vi "BlockDiagram.vi"(6 "error in":errorcluster, 9 "PythonConverter in":refnum<class "PythonBDConverter.lvclass">) -> (0 "error out":errorcluster, 3 "PythonConverter out":refnum<class "PythonBDConverter.lvclass">, 4 "BlockDiagram":string)   [LabVIEW 2014, in "PythonBDConverter.lvclass"]
uses:
  PythonBDConverter.lvclass
  PythonBDConverter.lvclass/PythonBDConverter.ctl
  VI Interpreter/Classes/TopLevelDiagram/TopLevelDiagram.lvclass
  Parsing/Python Functions.lvlib
  VI Interpreter/Classes/VI Interpreter/VI Interpreter.lvclass
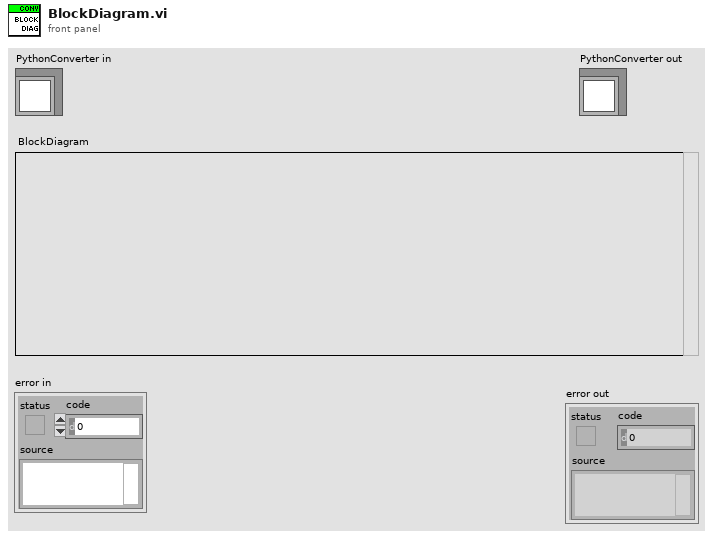
[diagram p1: front panel]
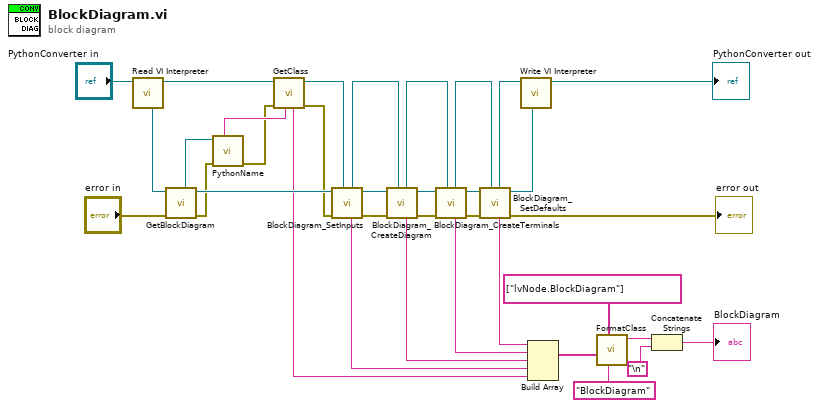
[diagram p0: block diagram]
diagram:
  n1 = call "Read VI Interpreter.vi"("PythonConverter_BD in"="PythonConverter in") -> ("PythonConverter_BD out"=w4:refnum<class "PythonBDConverter.lvclass">, "VI Interpreter"=w6:refnum<class "VI Interpreter.lvclass">)  [unwired: 7 in]
  n2 = call "GetBlockDiagram.vi"("error in"="error in", "VI Interpreter in"=w6) -> ("error out"=w10:errorcluster, "VI Interpreter out"=w14:refnum<class "VI Interpreter.lvclass">, "TopLevelDiagram"=w12:refnum<class "TopLevelDiagram.lvclass">)  [unwired: 5 in]
  n3 = call-dynamic "PythonName.vi"("error in"=w10, "Diagram in"=w12) -> ("error out"=w7:errorcluster, "UID"=w11:string)  [unwired: 6 in, 2 out]
  n4 = call "GetClass.vi"("name"=w11, "error in"=w7, "PythonConverter in"=w4) -> ("error out"=w8:errorcluster, "PythonConverter out"=w15:refnum<class "PythonBDConverter.lvclass">, "class"=w9:string)  [unwired: 4 in]
  n5 = call "BlockDiagram_SetInputs.vi"("PythonConverter in"=w15, "error in"=w8, "VI Interpreter in"=w14) -> ("error out"=w21:errorcluster, "VI Interpreter out"=w22:refnum<class "VI Interpreter.lvclass">, "set_inputs"=w20:string, "PythonConverter out"=w19:refnum<class "PythonBDConverter.lvclass">)  [unwired: 5 in]
  n6 = call "BlockDiagram_CreateDiagram.vi"("PythonConverter in"=w19, "error in"=w21, "VI Interpreter in"=w22) -> ("error out"=w24:errorcluster, "VI Interpreter out"=w26:refnum<class "VI Interpreter.lvclass">, "create_diagram"=w25:string, "PythonConverter out"=w18:refnum<class "PythonBDConverter.lvclass">)  [unwired: 5 in]
  n7 = call "BlockDiagram_CreateTerminals.vi"("PythonConverter in"=w18, "error in"=w24, "VI Interpreter in"=w26) -> ("error out"=w23:errorcluster, "VI Interpreter out"=w28:refnum<class "VI Interpreter.lvclass">, "create_terminals"=w27:string, "PythonConverter out"=w17:refnum<class "PythonBDConverter.lvclass">)  [unwired: 5 in]
  n8 = call "BlockDiagram_SetDefaults.vi"("PythonConverter in"=w17, "error in"=w23, "VI Interpreter in"=w28) -> ("error out"=→"error out":errorcluster, "VI Interpreter out"=w3:refnum<class "VI Interpreter.lvclass">, "set_defaults"=w29:string, "PythonConverter out"=w2:refnum<class "PythonBDConverter.lvclass">)  [unwired: 5 in]
  n9 = call "Write VI Interpreter.vi"("VI Interpreter"=w3, "PythonConverter_BD in"=w2) -> ("PythonConverter_BD out"=→"PythonConverter out":refnum<class "PythonBDConverter.lvclass">)  [unwired: 7 in]
  n10 = Build Array(w29, w27, w25, w20, w9) -> (w33:string[])
  n11 = call "FormatClass.vi"("name"="BlockDiagram", "parameters/ancestors"=string[] ["lvNode.BlockDiagram"], "body"=w33) -> ("python"=w34:string)  [unwired: 8 in]
  n12 = Concatenate Strings(w34, "\n") -> (→"BlockDiagram":string)
